vi "Get Frame Position (Index).vi"(8 "error in (no error)":errorcluster, 11 "Reader in":refnum<class "Reader.lvclass">) -> (0 "error out":errorcluster, 3 "Reader":refnum<class "Reader.lvclass">)   [LabVIEW 2020, in "video_io.lvlib" / "Reader.lvclass"]
uses:
  Reader.lvclass
  Reader.lvclass/Reader.ctl
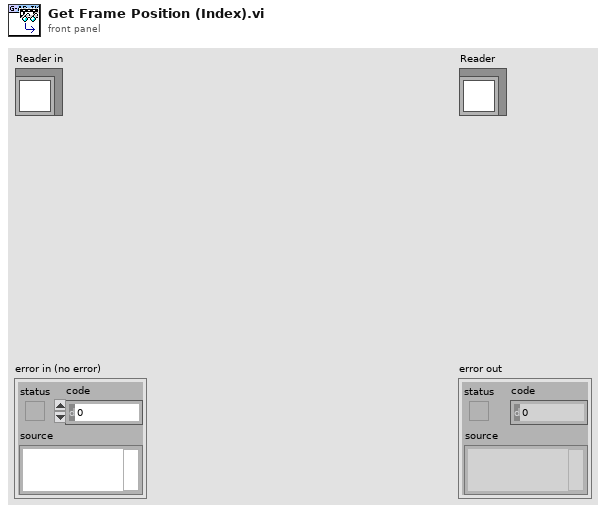
[diagram p1: front panel]
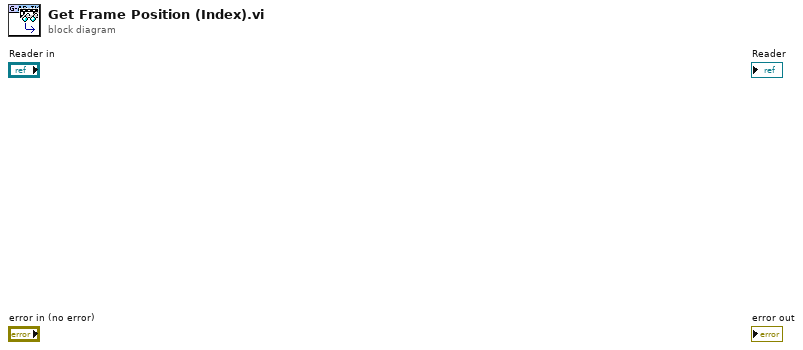
[diagram p0: block diagram]
diagram:
